vi "configure assembly.vi"(8 "error in":errorcluster, 10 "assembly definition in":T2={"name"="", "Instance ID"=100, "Type"=enum."Producing", "Size (elements)"=32, "big endian?"=FALSE, "data type"=enum."Double"}, 11 "EthernetIP configuration":refnum<class "EthernetIP configuration.lvclass">) -> (0 "error out":errorcluster, 1 "success":bool, 2 "assembly definition out":T2={"name"="", "Instance ID"=100, "Type"=enum."Producing", "Size (elements)"=32, "big endian?"=FALSE, "data type"=enum."Double"}, 5 "changed":bool)   [LabVIEW 2013, in "EthernetIP editor node.lvclass"]
uses:
  EthernetIP editor node.lvclass
  configuration/EthernetIP configuration.lvclass
  configuration/assembly type.ctl
  configuration/assembly definition.ctl
  <vilib>/NI/Tag Bus/tag/Data Type.ctl
  <vilib>/NI/Tag Bus/tag/tag descriptor.lvclass
panel:
  in  "Data Type":i32(listbox)
  in  "byte order":enum32{"Little", "Big"}(radio)
  in  "Elements":u32
  in  "Instance ID":u32
  in  "Asm Type":T1
  in  "Assembly Name (opt)":string
  in  "cancel":bool
  in  "ok":bool
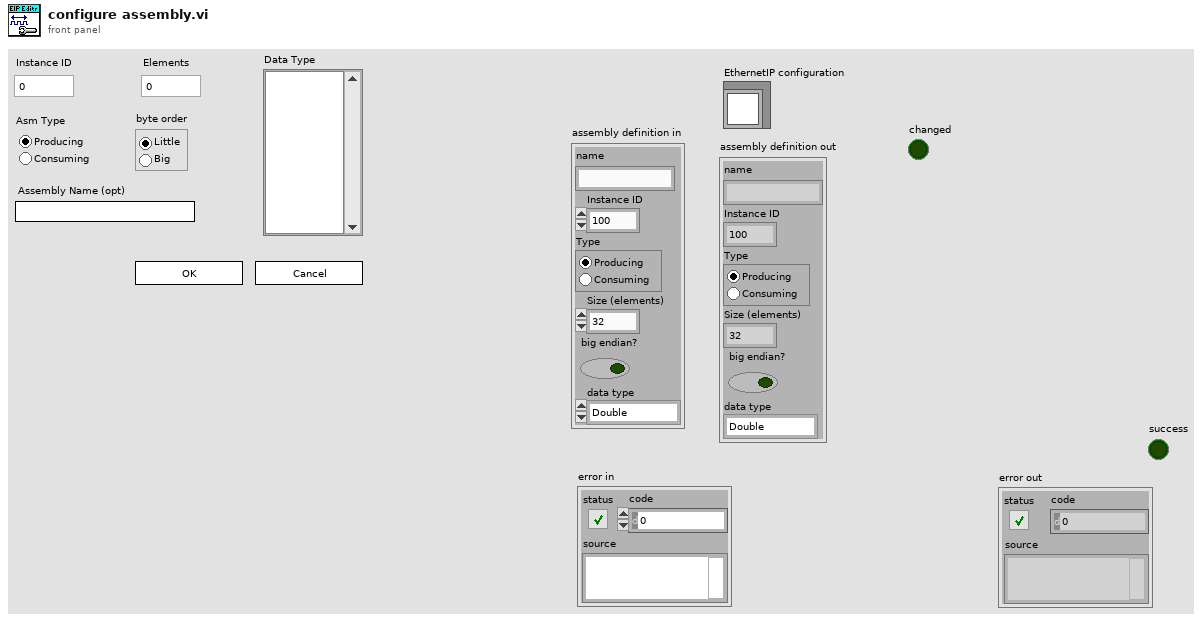
[diagram p1: front panel]
types:
  T1 = typedef "EthernetIP configuration.lvclass/assembly type.ctl" = enum32{"Producing", "Consuming"}
  T2 = typedef "EthernetIP configuration.lvclass/assembly definition.ctl" = cluster{"name":string, "Instance ID":u32, "Type":T1, "Size (elements)":u32, "big endian?":bool, "data type":T3}
  T3 = typedef "tag bus.lvlib/tag descriptor.lvclass/Data Type.ctl" = enum16{"Double", "Single", "I64", "I32", "I16", "I8", "U64", "U32", "U16", "U8", "Boolean", "String", "Array of Double", "Array of Single", "Array of I64", "Array of I32", "Array of I16", "Array of I8", "Array of U64", "Array of U32", "Array of U16", "Array of U8", "Array of Boolean", "Array of String"}
  T4 = enum32{"Invalid", "Standard", "Closed", "Hidden", "Minimized", "Maximized"}
  T5 = enum32{"Invalid", "Default", "Floating", "Floating/Auto-Hide", "Modal"}
  T6 = enum32{"invalid app kind", "Development System", "Run Time System", "Student Edition", "Embedded LabVIEW", "Evaluation", "Custom"}
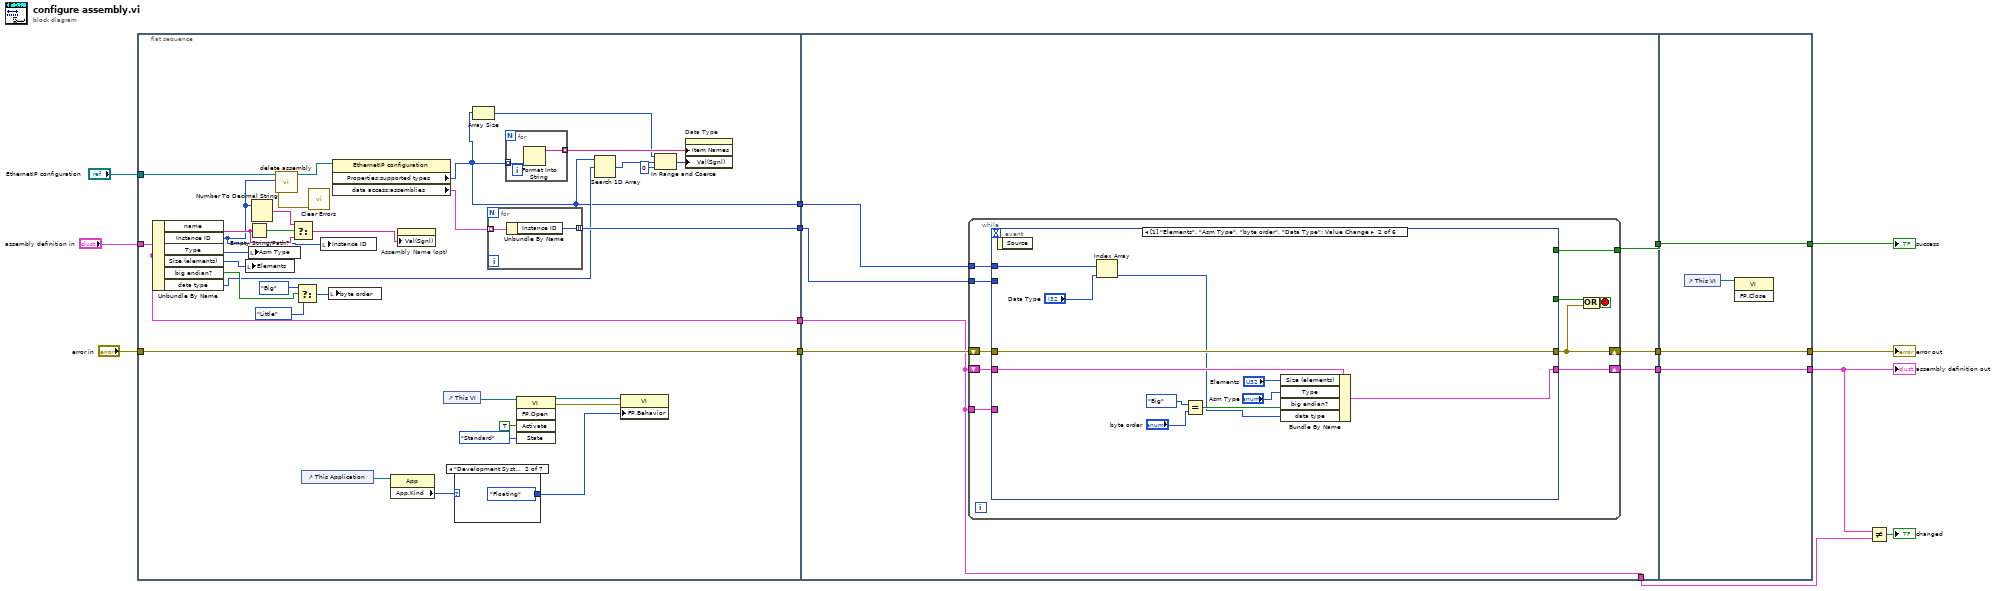
[diagram p0: block diagram]
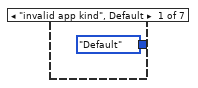
[diagram p2: hidden frame]
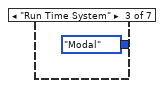
[diagram p3: hidden frame]
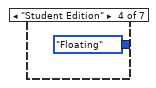
[diagram p4: hidden frame]
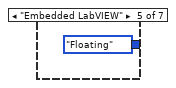
[diagram p5: hidden frame]
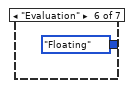
[diagram p6: hidden frame]
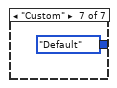
[diagram p7: hidden frame]
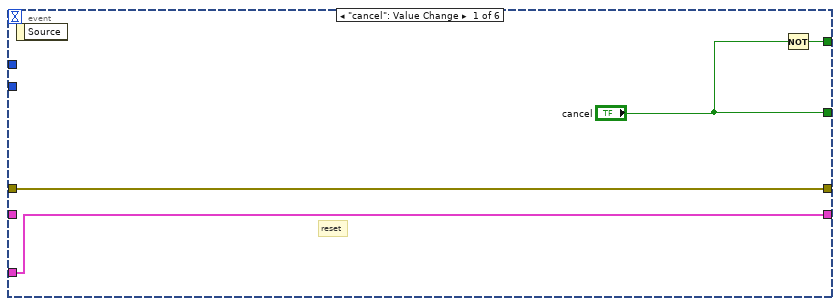
[diagram p8: hidden frame]
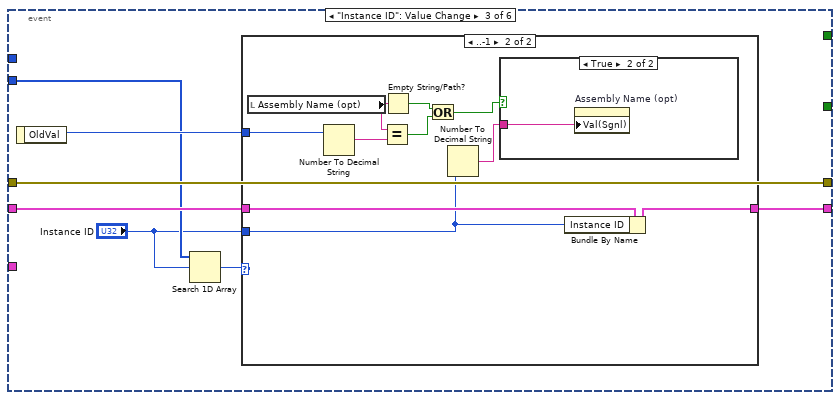
[diagram p9: hidden frame]
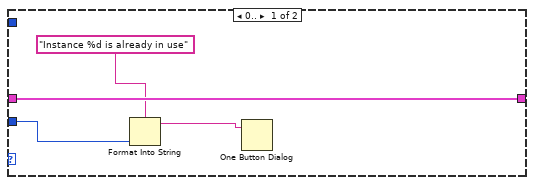
[diagram p10: hidden frame]
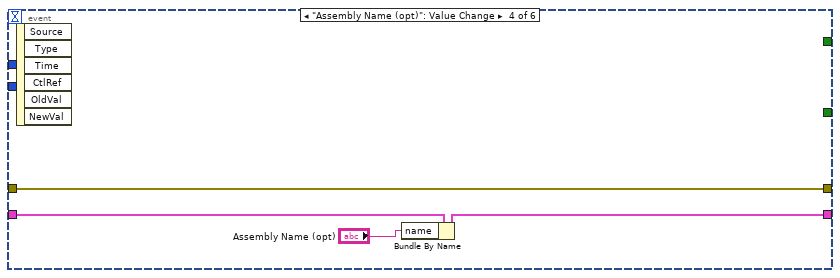
[diagram p12: hidden frame]
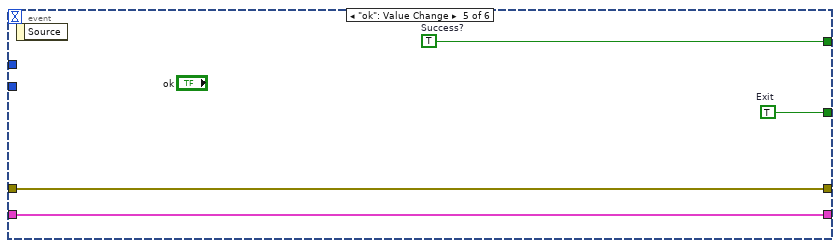
[diagram p13: hidden frame]
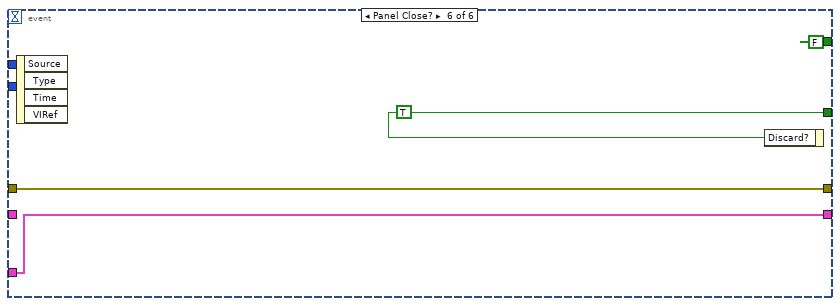
[diagram p14: hidden frame]
diagram:
  n1 = flat-sequence {
    tunnel: "error in" -> [w32]
    tunnel: "EthernetIP configuration" -> [w40]
    tunnel: "assembly definition in" -> [w28]
    tunnel: [w36] -> w6
    tunnel: [w32] -> w5
    tunnel: [w28] -> w4
    tunnel: [w18] -> w1
    tunnel: [w66] -> w11
    tunnel: [w65] -> w10
    tunnel: [w64] -> w9
    tunnel: w6 -> [w61]
    tunnel: w5 -> [w63]
    tunnel: w4 -> [w62]
    tunnel: [w62] -> w3
    tunnel: w1 -> [w60]
    tunnel: [w127] -> w2
    tunnel: [w128] -> w13
    tunnel: [w129] -> w14
    tunnel: w11 -> [w129]
    tunnel: w10 -> [w128]
    tunnel: w9 -> [w127]
    frame #0 {
      n2 = Unbundle By Name(w28) -> ("name"=w34:string, "Instance ID"=w30:u32, "Type"=w31:T1, "Size (elements)"=w29:u32, "big endian?"=w23:bool, "data type"=w20:T3)
      n3 = local write "Elements"(w29) -> ()
      n4 = local write "Asm Type"(w31) -> ()
      n5 = Empty String/Path?(string/path=w34) -> (empty?=w35:bool)
      n6 = Number To Decimal String(number=w30) -> (decimal integer string=w33:string)  [unwired: 1 in]
      n7 = call "delete assembly.vi"("instance ID"=w30, "EthernetIP configuration in"=w40) -> ("error out"=w37:errorcluster, "EthernetIP configuration out"=w38:refnum<class "EthernetIP configuration.lvclass">)  [unwired: 7 in, 1 out]
      n8 = Select(t=w33, s=w35, f=w34) -> (s? t:f=w27:string)
      n9 = Select(t=enum32{"Little", "Big"}."Big" ("byte order"), s=w23, f=enum32{"Little", "Big"}."Little" ("byte order")) -> (s? t:f=w24:enum32{"Little", "Big"})
      n10 = control-ref of="This Application"() -> (w43:refnum<vi>)
      n11 = call <vilib>:"Clear Errors.vi"("error in (no error)"=w37) -> ()  [unwired: 6 in, 1 out]
      n12 = local write "Instance ID"(w30) -> ()
      n13 = local write "byte order"(w24) -> ()
      n14 = property class="EthernetIP configuration"(reference=w38) -> ("Properties:supported types"=w18:T3[], "data access:assemblies"=w39:T2[])  [unwired: 1 in, 2 out]
      n15 = property class="App"(reference=w43) -> ("App.Kind"=w42:T6)  [unwired: 1 in, 2 out]
      n16 = property on="Assembly Name (opt)" class="Str"("Val(Sgnl)"=w27) -> ()  [unwired: 2 in, 2 out]
      n17 = control-ref of="This VI"() -> (w44:refnum<vi>)
      n18 = case shown="\"Development System\"" w42 {
        tunnel: [T5."Default" ("Front Panel Window:Behavior") T5."Floating" ("Front Panel Window:Behavior") T5."Modal" ("Front Panel Window:Behavior") T5."Floating" ("Front Panel Window:Behavior") T5."Floating" ("Front Panel Window:Behavior") T5."Floating" ("Front Panel Window:Behavior") T5."Default" ("Front Panel Window:Behavior")] -> w41
        frame "invalid app kind", Default {
        }
        frame "Development System" {
        }
        frame "Run Time System" {
        }
        frame "Student Edition" {
        }
        frame "Embedded LabVIEW" {
        }
        frame "Evaluation" {
        }
        frame "Custom" {
        }
      }
      n19 = Array Size(array=w18) -> (size(s)=w17:i32)
      n20 = for {
        tunnel: w39 -> [w52] mode=indexing
        tunnel: [w51] -> w36 mode=indexing
        n21 = Unbundle By Name(w52) -> ("Instance ID"=w51:u32)
      }
      n22 = for {
        tunnel: w18 -> [w50] mode=indexing
        tunnel: [w49] -> w22 mode=indexing
        n23 = Format Into String(w50) -> (resulting string=w49:string)  [unwired: 3 in, 1 out]
      }
      n24 = invoke class="VI" method="FP.Open"(reference=w44, "Activate"=TRUE ("Activate?"), "State"=T4."Standard") -> (reference out=w47:refnum<vi>, error out=w48:errorcluster)  [unwired: 2 in, 3 out]
      n25 = Search 1D Array(1D array=w18, element=w20) -> (index of element=w21:i32)  [unwired: 1 in]
      n26 = property class="VI"(reference=w47, error in=w48, "FP.Behavior"=w41) -> ()  [unwired: 2 out]
      n27 = In Range and Coerce(upper limit=w17, x=w21, lower limit=0) -> (coerced(x)=w19:i32)  [unwired: 1 out]
      n28 = property on="Data Type" class="LstBox (strict)"("Item Names"=w22, "Val(Sgnl)"=w19) -> ()  [unwired: 2 in, 2 out]
    }
    frame #1 {
      n29 = while {
        shift-right: [w71] -> w65
        shift-left: w63 -> [w76]
        tunnel: [w75] -> w66
        shift-right: [w69] -> w64
        shift-left: w62 -> [w72]
        tunnel: w62 -> [w70]
        tunnel: w61 -> [w68]
        tunnel: w60 -> [w67]
        stop <- w73 stop-if-true
        n30 = event shown="[1] \"Elements\", \"Asm Type\", \"byte order\", \"Data Type\": Value Change" {
          selector: _ -> [_ _ _ _ _ _]
          dyn-events: _ -> [_ _ _ _ _ _]
          timeout: _ -> [_ _ _ _ _ _]
          tunnel: w76 -> [w80 w91 w98 w117 w121 w125]
          tunnel: [w80 w91 w98 w117 w121 w125] -> w71
          tunnel: [w79 _ _ _ w118 FALSE] -> w75
          tunnel: ["cancel" _ _ _ w119 w123] -> w74
          tunnel: w72 -> [_ w90 w97 w116 w120 _]
          tunnel: [w77 w89 w96 w115 w120 w122] -> w69
          tunnel: w70 -> [w77 _ _ _ _ w122]
          tunnel: w68 -> [_ _ w94 _ _ _]
          tunnel: w67 -> [_ w83 _ _ _ _]
          event "cancel": Value Change {
            # "reset"
            n31 = event-data() -> ()  [unwired: 1 in, 1 out]
            n32 = Not(x="cancel") -> (.not. x?=w79:bool)
          }
          event "Elements", "byte order", "Data Type": Value Change {
            n33 = event-data() -> ()  [unwired: 1 in, 1 out]
            n34 = Index Array(array=w83, index="Data Type") -> (element=w81:T3)
            n35 = Equal?(x=enum32{"Little", "Big"}."Big" ("byte order"), y="byte order") -> (x = y?=w84:bool)
            n36 = Bundle By Name(cluster=w90, "Size (elements)"="Elements", "Type"="Asm Type", "big endian?"=w84, "data type"=w81) -> (w89:T2)
          }
          event "Instance ID": Value Change {
            n37 = event-data() -> ("OldVal"=w95:u32)  [unwired: 1 in]
            n38 = Search 1D Array(1D array=w94, element="Instance ID") -> (index of element=w92:i32)  [unwired: 1 in]
            n39 = case shown="..-1" w92 {
              tunnel: w97 -> [w102 w112]
              tunnel: [w102 w111] -> w96
              tunnel: w95 -> [_ w110]
              tunnel: "Instance ID" -> [w101 w103]
              frame 0.. {
                n40 = Format Into String(format string="Instance %d is already in use", w101) -> (resulting string=w100:string)  [unwired: 2 in, 1 out]
                n41 = One Button Dialog(message=w100) -> ()  [unwired: 1 in, 1 out]
              }
              frame ..-1 {
                n42 = local read "Assembly Name (opt)"() -> (w106:string)
                n43 = Number To Decimal String(number=w110) -> (decimal integer string=w107:string)  [unwired: 1 in]
                n44 = Equal?(x=w106, y=w107) -> (x = y?=w108:bool)
                n45 = Empty String/Path?(string/path=w106) -> (empty?=w109:bool)
                n46 = Or(x=w109, y=w108) -> (x .or. y?=w105:bool)
                n47 = Number To Decimal String(number=w103) -> (decimal integer string=w104:string)  [unwired: 1 in]
                n48 = case shown="True" w105 {
                  tunnel: w104 -> [_ w113]
                  frame False {
                  }
                  frame True {
                    n49 = property on="Assembly Name (opt)" class="Str"("Val(Sgnl)"=w113) -> ()  [unwired: 2 in, 2 out]
                  }
                }
                n50 = Bundle By Name(cluster=w112, "Instance ID"=w103) -> (w111:T2)
              }
            }
          }
          event "Assembly Name (opt)": Value Change {
            n51 = event-data() -> ()  [unwired: 1 in, 6 out]
            n52 = Bundle By Name(cluster=w116, "name"="Assembly Name (opt)") -> (w115:T2)
          }
          event "ok": Value Change {
            w118 = TRUE  # Success?
            w119 = TRUE  # Exit
            n53 = event-data() -> ()  [unwired: 1 in, 1 out]
          }
          event Panel Close? {
            w123 = TRUE ("cancel")
            n54 = event-data() -> ()  [unwired: 1 in, 4 out]
            n55 = event-data("Discard?"=w123) -> ()  [unwired: 1 in, 1 out]
          }
        }
        n56 = Compound Arithmetic op=OR(w74, w71) -> (w73:bool)
      }
    }
    frame #2 {
      n57 = control-ref of="This VI"() -> (w126:refnum<vi>)
      n58 = invoke class="VI" method="FP.Close"(reference=w126) -> ()  [unwired: 2 in, 3 out]
    }
  }
  n59 = Not Equal?(x=w2, y=w3) -> (x != y?=→"changed":bool)
  "error out" <- w13
  "success" <- w14
  "assembly definition out" <- w2
